vi "Keyence.Main.Status.vi"(7 "Idx":i32, 8 "error in":errorcluster, 11 "Data in":T1={"Status"={"State"=enum."Init", "Ref"=refnum, "Bank"=0, "Version"="", "Model"="", "EndTS"=timestamp(0 s since 1904-01-01), "ImgPath"=path "", "Tuned"=FALSE}, "Sets"={"IP"="192.168.2.1", "Timeout_ms"=5000, "Retries"=0, "ReconnectPeriod_s"=0, "ResetPeriod_s"=0, "ReadImg"=FALSE}, "Code"={"text"="", "status"=FALSE, "corners"=[], "level"=0, "class"="", "path"=path ""}}) -> (0 "error out":errorcluster, 3 "Data out":T1={"Status"={"State"=enum."Init", "Ref"=refnum, "Bank"=0, "Version"="", "Model"="", "EndTS"=timestamp(0 s since 1904-01-01), "ImgPath"=path "", "Tuned"=FALSE}, "Sets"={"IP"="192.168.2.1", "Timeout_ms"=5000, "Retries"=0, "ReconnectPeriod_s"=0, "ResetPeriod_s"=0, "ReadImg"=FALSE}, "Code"={"text"="", "status"=FALSE, "corners"=[], "level"=0, "class"="", "path"=path ""}})   [LabVIEW 2016]
uses:
  Keyence.Data.ctl
  Keyence.Data.Status.ctl
  Keyence.Data.Status.State.ctl
  Keyence.Data.Sets.ctl
  LowLevel/Keyence.CodeDetails.ctl
  tools/EventLog/EventLog.EventSource.ctl
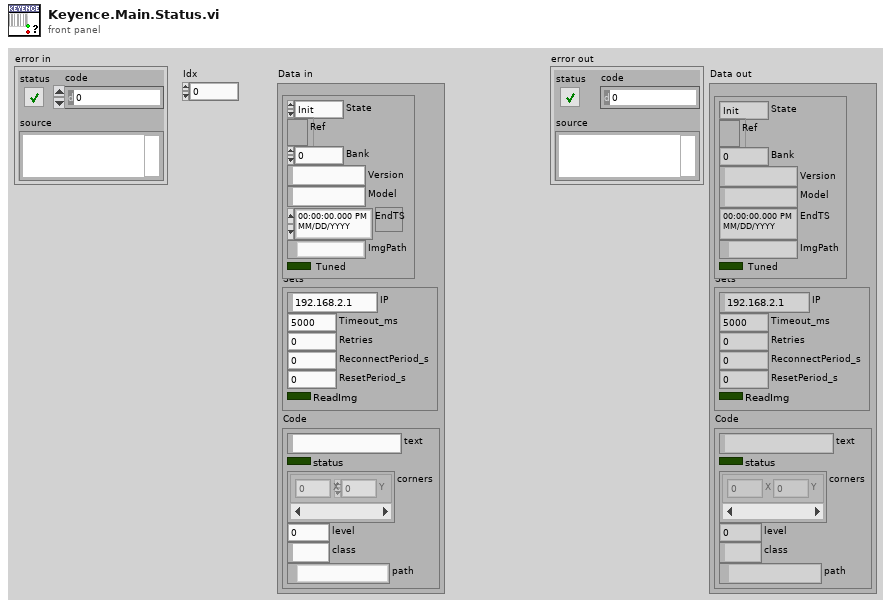
[diagram p1: front panel]
types:
  T1 = typedef "Keyence.Data.ctl" = cluster{"Status":T2, "Sets":T4, "Code":T5}
  T2 = typedef "Keyence.Data.Status.ctl" = cluster{"State":T3, "Ref":refnum<k5>, "Bank":u8, "Version":string, "Model":string, "EndTS":timestamp, "ImgPath":path, "Tuned":bool}
  T3 = typedef "Keyence.Data.Status.State.ctl" = enum16{"First", "Init", "Reset", "Idle", "Scan", "Tune"}
  T4 = typedef "Keyence.Data.Sets.ctl" = cluster{"IP":string, "Timeout_ms":i32, "Retries":i32, "ReconnectPeriod_s":i32, "ResetPeriod_s":i32, "ReadImg":bool}
  T5 = typedef "Keyence.CodeDetails.ctl" = cluster{"text":string, "status":bool, "corners":cluster{"X":i32, "Y":i32}[], "level":u8, "class":string, "path":path}
  T6 = typedef "EventLog.EventSource.ctl" = enum16{"All", "Gui", "Ref", "File", "Arch", "Seq", "CPX", "DB", "Laser", "Scan.P", "Scan.O"}
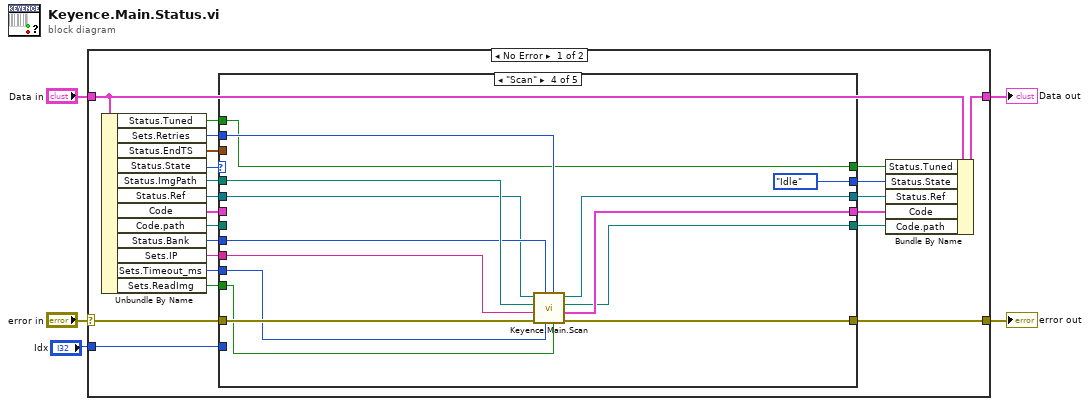
[diagram p0: block diagram]
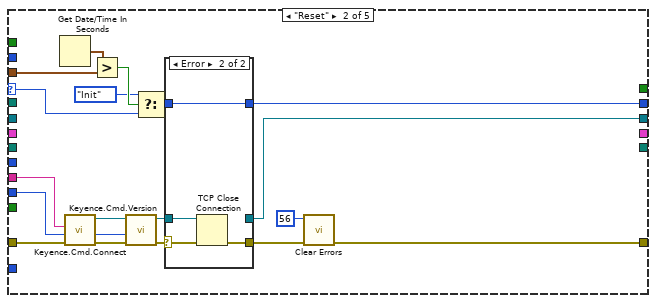
[diagram p3: hidden frame]
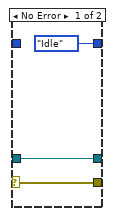
[diagram p4: hidden frame]
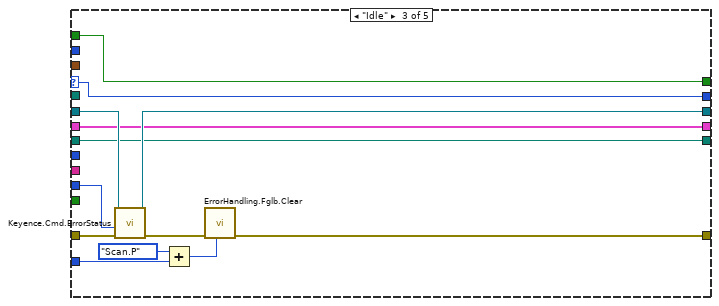
[diagram p5: hidden frame]
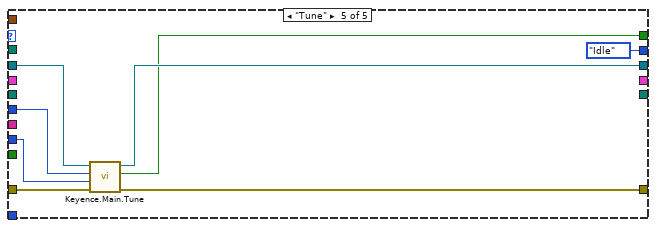
[diagram p6: hidden frame]
diagram:
  n1 = case shown="No Error" "error in" {
    selector: "error in" -> [w25 w92]
    tunnel: [w20 w92] -> w2
    tunnel: "Data in" -> [w26 w91]
    tunnel: [w27 w91] -> w3
    tunnel: "Idx" -> [w10 _]
    frame No Error {
      n2 = Unbundle By Name(w26) -> ("Status.Tuned"=w7:bool, "Sets.Retries"=w17:i32, "Status.EndTS"=w18:timestamp, "Status.State"=w22:T3, "Status.ImgPath"=w9:path, "Status.Ref"=w24:refnum<k5>, "Code"=w14:T5, "Code.path"=w12:path, "Status.Bank"=w16:u8, "Sets.IP"=w23:string, "Sets.Timeout_ms"=w21:i32, "Sets.ReadImg"=w13:bool)
      n3 = case shown="\"Scan\"" w22 {
        selector: w22 -> [w29 w33 w56 _ _]
        tunnel: w25 -> [w28 w48 w67 w78 w90]
        tunnel: [w28 w41 w68 w79 w89] -> w20
        tunnel: w24 -> [w30 _ w65 w73 w88]
        tunnel: w23 -> [_ w32 _ w70 _]
        tunnel: w21 -> [_ w40 w64 w74 w85]
        tunnel: [w29 w39 w56 Keyence.Data.Status.State."Idle" ("State") Keyence.Data.Status.State."Idle" ("State")] -> w19
        tunnel: w18 -> [_ w38 _ _ _]
        tunnel: w17 -> [_ _ _ w81 _]
        tunnel: w16 -> [_ _ _ w75 w87]
        tunnel: [_ _ w62 w72 _] -> w15
        tunnel: w14 -> [_ _ w62 _ _]
        tunnel: w13 -> [_ _ _ w69 _]
        tunnel: [_ _ w61 w71 _] -> w11
        tunnel: w12 -> [_ _ w61 _ _]
        tunnel: w10 -> [_ _ w59 _ _]
        tunnel: w9 -> [_ _ _ w77 _]
        tunnel: [w30 w31 w66 w82 w84] -> w8
        tunnel: [_ _ w57 w76 w83] -> w6
        tunnel: w7 -> [_ _ w57 w76 _]
        frame "First", "Init" {
        }
        frame "Reset" {
          n4 = Get Date/Time In Seconds() -> (seconds since 1Jan1904=w37:timestamp)
          n5 = call "Keyence.Cmd.Connect.vi"("error in (no error)"=w48, "Timeout [ms] (1000)"=w40, "IP"=w32) -> ("error out"=w47:errorcluster, "connection ID out"=w46:refnum<k5>)  [unwired: 7 in]
          n6 = Greater?(x=w37, y=w38) -> (0:w36:bool)
          n7 = call "Keyence.Cmd.Version.vi"("error in (no error)"=w47, "Timeout [ms] (1000)"=w40, "connection ID"=w46) -> ("error out"=w45:errorcluster, "connection ID out"=w44:refnum<k5>)  [unwired: 4 in, 3 out]
          n8 = Select(t=Keyence.Data.Status.State."Init" ("f"), s=w36, f=w33) -> (s? t:f=w35:T3)
          n9 = case shown="Error" w45 {
            selector: w45 -> [w51 w55]
            tunnel: w44 -> [w50 w54]
            tunnel: [w51 w53] -> w42
            tunnel: [w50 _] -> w31
            tunnel: [Keyence.Data.Status.State."Idle" ("Status.State") w52] -> w39
            tunnel: w35 -> [_ w52]
            frame No Error {
            }
            frame Error {
              n10 = TCP Close Connection(connection ID=w54, error in (no error)=w55) -> (error out=w53:errorcluster)  [unwired: 1 in, 1 out]
            }
          }
          n11 = call <vilib>:"Clear Errors.vi"("error in (no error)"=w42, "specific error code to clear (0: all)"=56) -> ("error out"=w41:errorcluster)  [unwired: 4 in, 1 out]
        }
        frame "Idle" {
          n12 = call "Keyence.Cmd.ErrorStatus.vi"("error in (no error)"=w67, "Timeout [ms] (1000)"=w64, "connection ID"=w65) -> ("error out"=w63:errorcluster, "connection ID out"=w66:refnum<k5>)  [unwired: 5 in, 2 out]
          n13 = Add(x=EventLog.EventSource."Scan.P" ("Event source"), y=w59) -> (x+y=w58:i32)
          n14 = call "ErrorHandling.Fglb.Clear.vi"("Event source"=w58, "error in (no error)"=w63) -> ("error out"=w68:errorcluster)  [unwired: 9 in]
        }
        frame "Scan" {
          n15 = call "Keyence.Main.Scan.vi"("ReadImg"=w69, "Retries"=w81, "Timeout_ms"=w74, "Bank"=w75, "error in (no error)"=w78, "IP"=w70, "ImgPath"=w77, "TCP Network Connection in"=w73) -> ("error out"=w79:errorcluster, "Code"=w72:T5, "File name"=w71:path, "TCP Network Connection out"=w82:refnum<k5>)
        }
        frame "Tune" {
          n16 = call "Keyence.Main.Tune.vi"("error in (no error)"=w90, "Timeout_ms"=w85, "Bank"=w87, "TCP Network Connection in"=w88) -> ("error out"=w89:errorcluster, "Tune succeded"=w83:bool, "TCP Network Connection out"=w84:refnum<k5>)  [unwired: 5 in]
        }
      }
      n17 = Bundle By Name(cluster=w26, "Status.Tuned"=w6, "Status.State"=w19, "Status.Ref"=w8, "Code"=w15, "Code.path"=w11) -> (w27:T1)
    }
    frame Error {
    }
  }
  "error out" <- w2
  "Data out" <- w3
